vi "setWidth.vi"(8 "error in (no error)":errorcluster, 10 "width":i32, 11 "pRectangle in":refnum<class "pRectangle.lvclass">) -> (0 "error out":errorcluster, 3 "pRectangle out":refnum<class "pRectangle.lvclass">)   [LabVIEW 2018, in "pRectangle.lvclass"]
uses:
  pRectangle.lvclass
  pRectangle.lvclass/pRectangle.ctl
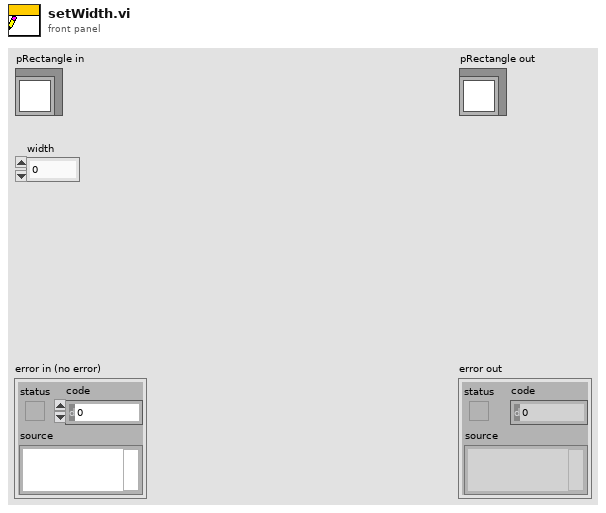
[diagram p1: front panel]
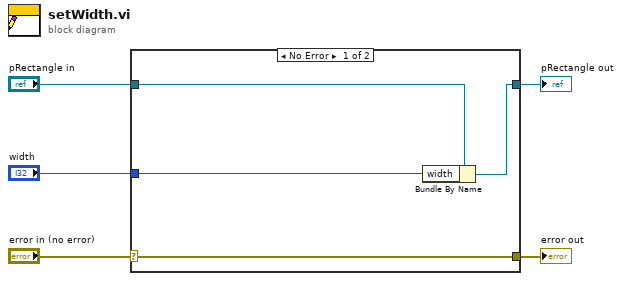
[diagram p0: block diagram]
diagram:
  n1 = case shown="No Error" "error in (no error)" {
    selector: "error in (no error)" -> [w9 w10]
    tunnel: [w9 w10] -> w4
    tunnel: [w7 w11] -> w2
    tunnel: "pRectangle in" -> [w8 w11]
    tunnel: "width" -> [w6 _]
    frame No Error {
      n2 = Bundle By Name(cluster=w8, "width"=w6) -> (w7:refnum<class "pRectangle.lvclass">)
    }
    frame Error {
    }
  }
  "error out" <- w4
  "pRectangle out" <- w2
